vi "Config.vi"(8 "error in (no error)":errorcluster, 10 "Setting":T1={"Freq"=1000.0, "Range"=enum."10m Ohm", "Measurements"=enum."Impedence"} {"Freq" min=0.1 max=1050.0 step=0.01 format="%_5e"}, 11 "ACIR in":refnum<class "ACIR.lvclass">) -> (0 "error out":errorcluster, 3 "ACIR out":refnum<class "ACIR.lvclass">)   [LabVIEW 2021, in "HAL.lvlib" / "ACIR.lvclass"]
uses:
  ACIR.lvclass
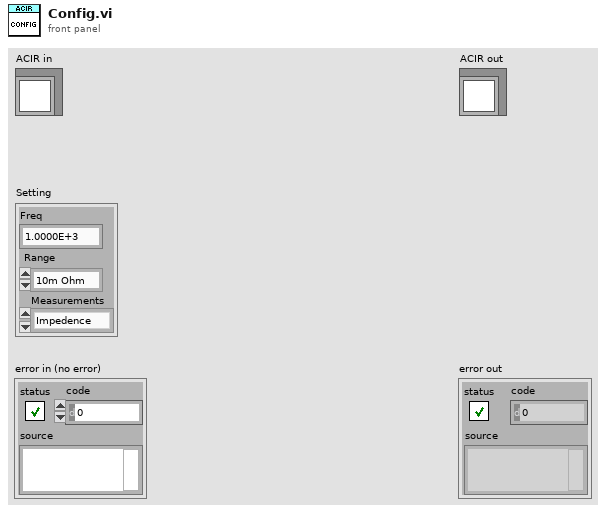
[diagram p1: front panel]
types:
  T1 = cluster{"Freq":dbl, "Range":enum16{"3m Ohm", "10m Ohm", "100m Ohm"}, "Measurements":enum16{"Impedence", "Phase Angle", "OCV"}}
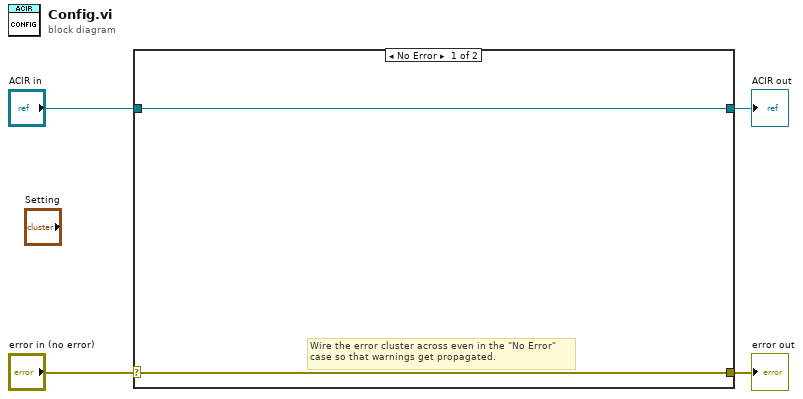
[diagram p0: block diagram]
diagram:
  n1 = case shown="No Error" "error in (no error)" {
    selector: "error in (no error)" -> [w5 w8]
    tunnel: [w5 w8] -> w3
    tunnel: [w6 w7] -> w1
    tunnel: "ACIR in" -> [w6 w7]
    frame No Error {
      # "Wire the error cluster across even in the \"No Error\"\ncase so that warnings get propagated."
    }
    frame Error {
    }
  }
  "error out" <- w3
  "ACIR out" <- w1
